vi "movment_practice.vi"() -> ()   [LabVIEW 2014]
uses:
  <vilib>/Motion/FlexMotion/CustomControls/CustomControls.llb/Axis To Control.flx
  <vilib>/Motion/FlexMotion/FunctionsVIs/StartStopMotion.llb/Start Motion (8 axes).flx
  <vilib>/Motion/FlexMotion/FunctionsVIs/Trajectory.llb/Check Move Complete Status (8 axes).flx
  <vilib>/Motion/FlexMotion/FunctionsVIs/StartStopMotion.llb/Stop Motion (8 axes).flx
panel:
  in  "stop 2":bool
  out "Waveform Chart 2":dynamicdata(graph)
  in  "Zero":dbl=-99.6 format="%#_13g"
  out "Waveform Chart":dynamicdata(graph)
  out "Force (grams)":dbl=0.3869919147841388
  in  "stop":bool
  out "Voltage (V)":dbl=0.3869919147841388
  out "Elapsed Time (s)":dbl format="%0.3f"
  out "Time from\nStart to finish (s)":dbl
  in  "FIRST - Motor":bool
  in  "Motor speed\nmm/s":dbl
  in  "distance to move\nmm (post to post)":dbl
  # "Outputs"
  # "Inputs"
  # "Both must be white\nto start program"
  # "To stop program,\npress both buttons"
  # "To feather the sample, let the sample first be slack and then keep in mind the voltage.\nThen put the sample in tension by only a small amount (~.001 volts), then stop the motor.\nIf the resting voltage is more than ~.001 volts higher than the initial voltage was, compress the sample\nRepeat until the sample is at its maximum resting length\n\nYou can similarly feather around a number if you're adjusting for a preload"
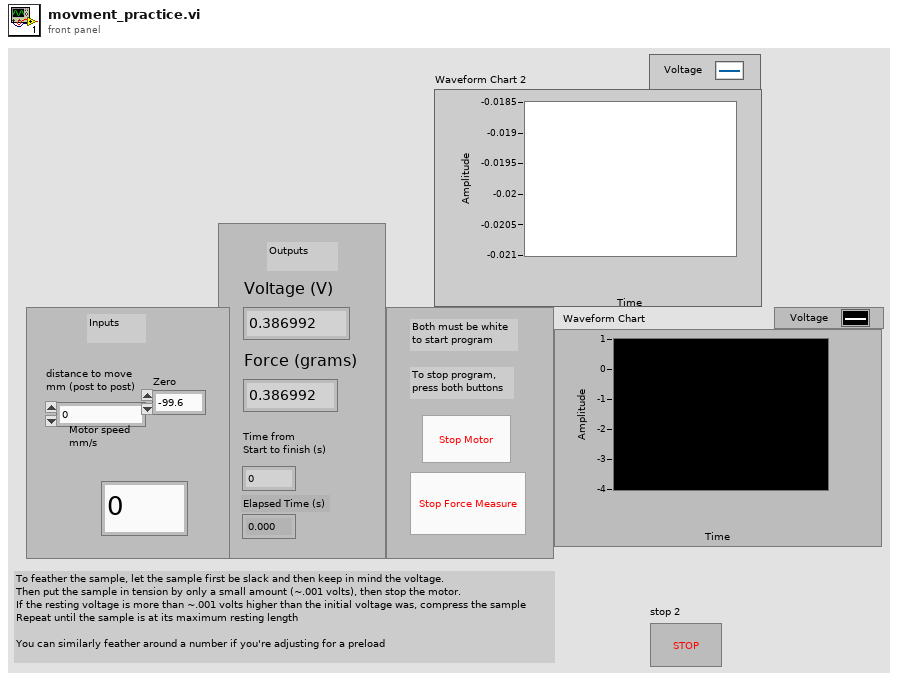
[diagram p1: front panel]
types:
  T1 = typedef "Board Id" = u8
  T2 = enum16{"Absolute Position", "Relative Position", "Velocity", "Relative to Cap Pos", "Modulus Position", "Absolute Contouring", "Relative Contouring"}
  T3 = typedef "Axis To Control.flx" = u16
  T4 = typedef "Resource Out (Enum).flx" = u16
  T5 = typedef "Bd Id Out" = u8
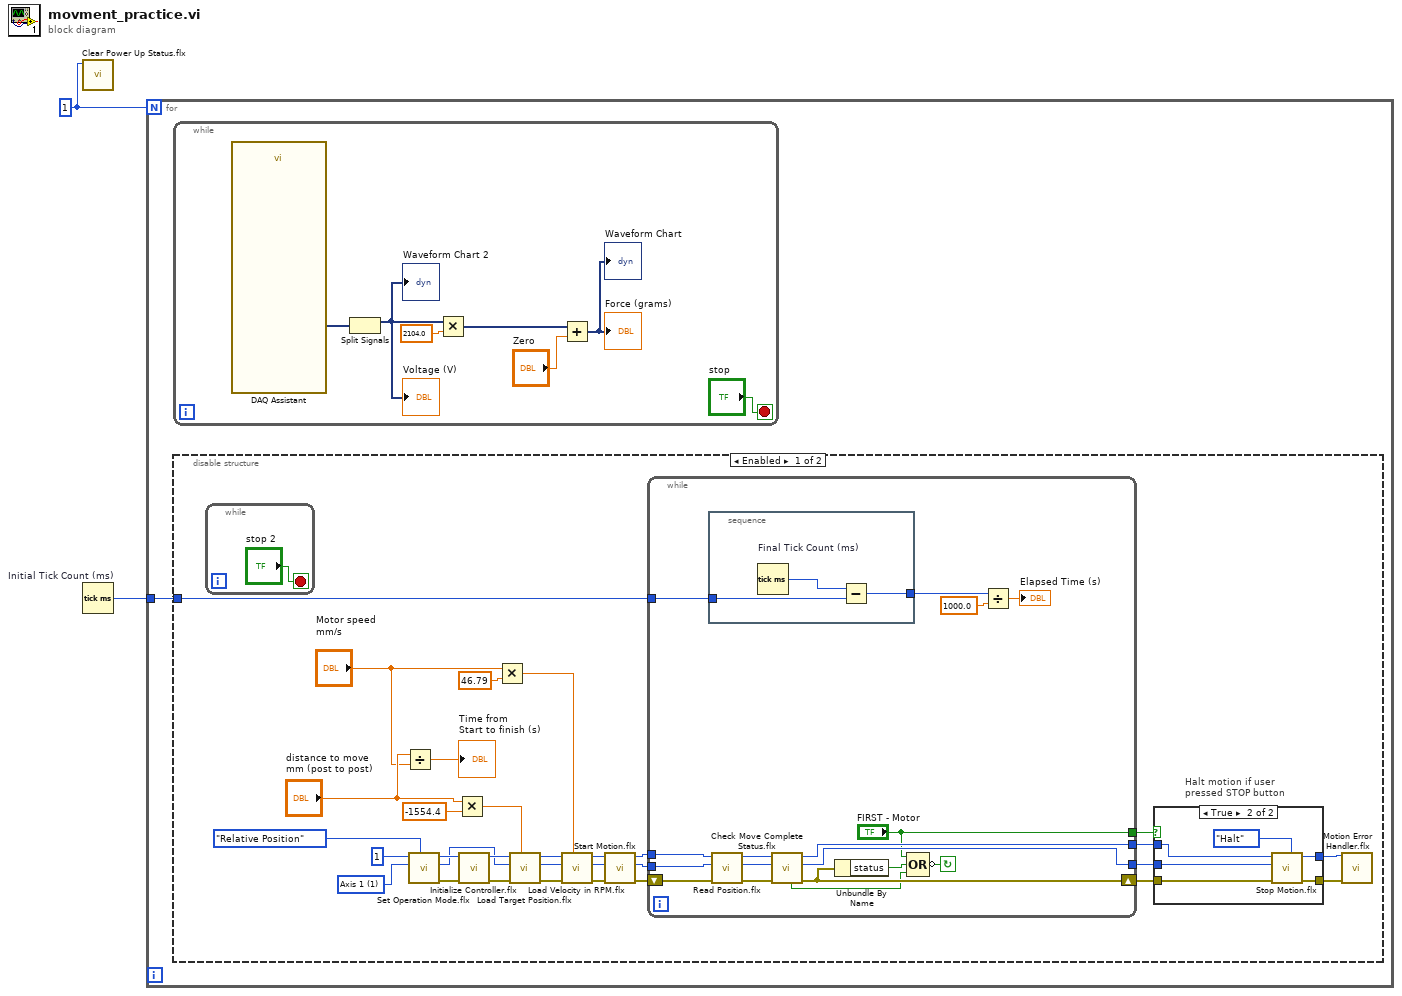
[diagram p0: block diagram]
diagram:
  w2 = 1
  n1 = call <vilib>:"Clear Power Up Status.flx"("Board ID"=w2) -> ()  [unwired: 6 in, 2 out]
  n2 = Tick Count (ms) "Initial Tick Count (ms)"() -> (millisecond timer value=w1:u32)
  n3 = for {
    N: w2 -> [_]
    tunnel: w1 -> [w3]
    n4 = while {
      stop <- "stop" stop-if-true
      n5 = call "DAQ Assistant"() -> ("data"=w9:dynamicdata)  [unwired: 16 in, 3 out]
      n6 = Split Signals(w9) -> (w4:dynamicdata)  [unwired: 2 in, 1 out]
      "Voltage (V)" <- w4
      "Waveform Chart 2" <- w4
      n7 = Multiply(x=w4, y=2104.0) -> (x*y=w8:dynamicdata)
      n8 = Add(x=w8, y="Zero") -> (x+y=→"Force (grams)" →"Waveform Chart":dynamicdata)
    }
    n9 = disable-structure shown="Enabled" {
      disable-tunnel: w3 -> [w14 _]
      frame Enabled {
        w31 = T3 1 items=["Axis 1"=1, "Axis 2"=2, "Axis 3"=3, "Axis 4"=4, "Axis 5"=5, "Axis 6"=6, "Axis 7"=7, "Axis 8"=8] ("Axis")
        # "Halt motion if user\npressed STOP button"
        n10 = while {
          stop <- "stop 2" stop-if-true
        }
        n11 = Divide(x="distance to move\nmm (post to post)", y="Motor speed\nmm/s") -> (x/y=→"Time from\nStart to finish (s)":dbl)
        n12 = call <vilib>:"Set Operation Mode.flx"("Position Mode (Absolute)"=T2."Relative Position", "Axis or Vector Space"=w31, "Board ID"=T1 1) -> ("error out"=w29:errorcluster, "Resource Output"=w11:T4, "Bd ID Out"=w28:T5)  [unwired: 3 in]
        n13 = Multiply(x="distance to move\nmm (post to post)", y=-1554.4) -> (x*y=w18:dbl)
        n14 = call <vilib>:"Initialize Controller.flx"("error in (no error)"=w29, "Board ID"=w28) -> ("error out"=w27:errorcluster, "Bd ID Out"=w26:T5)  [unwired: 6 in]
        n15 = Multiply(x="Motor speed\nmm/s", y=46.79) -> (x*y=w17:dbl)
        n16 = call <vilib>:"Load Target Position.flx"("Target Position (0)"=w18, "error in (no error)"=w27, "Axis"=w11, "Board ID"=w26) -> ("error out"=w39:errorcluster, "Resource Output"=w40:T4, "Bd ID Out"=w41:T5)  [unwired: 3 in]
        n17 = call <vilib>:"Load Velocity in RPM.flx"("Velocity (500)"=w17, "error in (no error)"=w39, "Axis or Vector Space"=w40, "Board ID"=w41) -> ("error out"=w32:errorcluster, "Resource Output"=w30:T4, "Bd ID Out"=w33:T5)  [unwired: 3 in]
        n18 = call-poly <vilib>:"Start Motion.flx"("error in (no error)"=w32, "Axis or Vector Space"=w30, "Board ID"=w33) -> ("error out"=w36:errorcluster, "Resource Output"=w35:T4, "Bd ID Out"=w34:T5)  [unwired: 3 in]
        n19 = while {
          tunnel: [w60] -> w20
          shift-left: w36 -> [w57]
          shift-right: [w61] -> w19
          tunnel: [w62] -> w21
          tunnel: w35 -> [w66]
          tunnel: w34 -> [w58]
          tunnel: w14 -> [w53]
          tunnel: ["FIRST - Motor"] -> w12
          stop <- w52 continue-if-true
          n20 = stacked-sequence {
            tunnel: w53 -> [w70]
            tunnel: [w68] -> w55
            frame #0 {
              n21 = Tick Count (ms) "Final Tick Count (ms)"() -> (millisecond timer value=w69:u32)
              n22 = Subtract(x=w69, y=w70) -> (x-y=w68:u32)
            }
          }
          n23 = call <vilib>:"Read Position.flx"("error in (no error)"=w57, "Axis"=w66, "Board ID"=w58) -> ("error out"=w64:errorcluster, "Resource Output"=w65:T4, "Bd ID Out"=w67:T5)  [unwired: 3 in, 1 out]
          n24 = call-poly <vilib>:"Check Move Complete Status.flx"("error in (no error)"=w64, "Axis or Vector Space"=w65, "Board ID"=w67) -> ("error out"=w61:errorcluster, "Resource Output"=w60:T4, "Bd ID Out"=w62:T5, "Move Complete"=w59:bool)  [unwired: 3 in]
          n25 = Unbundle By Name(w61) -> ("status"=w63:bool)
          n26 = Compound Arithmetic op=OR("FIRST - Motor", w63, w59) -> (invert w52:bool)
          n27 = Divide(x=w55, y=1000.0) -> (x/y=→"Elapsed Time (s)":dbl)
        }
        n28 = case shown="True" w12 {
          tunnel: w21 -> [w44 w49]
          tunnel: w19 -> [w43 w48]
          tunnel: [w43 w47] -> w25
          tunnel: [w44 w46] -> w24
          tunnel: w20 -> [_ w45]
          frame False {
          }
          frame True {
            n29 = call-poly <vilib>:"Stop Motion.flx"("Stop Type (Decel)"=enum16{"Decelerate", "Halt", "Kill"}."Halt", "error in (no error)"=w48, "Axis or Vector Space"=w45, "Board ID"=w49) -> ("error out"=w47:errorcluster, "Bd ID Out"=w46:T5)  [unwired: 3 in, 1 out]
          }
        }
        n30 = call <vilib>:"Motion Error Handler.flx"("Board ID"=w24, "error in (no error)"=w25) -> ()  [unwired: 9 in, 5 out]
      }
      frame Disabled {
      }
    }
  }
